vi "Launch NEW Window.vi"(5 "error in (no error)":errorcluster, 7 "Window Info":T1(array[cluster]), 8 "Window Type":T2, 9 "State Queue":string[](array[string])=["SC >>> Initialize"], 11 "wForms":waveform(dbl)[](array[waveform])) -> (19 "error OUT":errorcluster)   [LabVIEW 2020, in "SPWB.lvclass"]
uses:
  SPWB.lvclass
  Controls/Analysis Type.ctl
  API/GSwFormDSP_class/GSwFormDSP.lvclass
  <vilib>/addons/_AddQ/G#Object/G#Object.lvclass
panel:
  # "Please Wait ....\nOpening a NEW Window!"
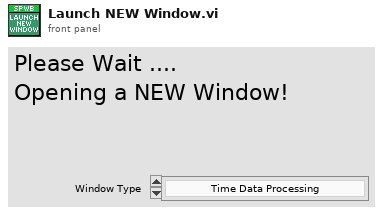
[diagram p1: front panel]
types:
  T1 = cluster{"Window Name Index":string, "wForm Ref":refnum<class "GSwFormDSP.lvclass">}[]
  T2 = typedef "SPWB.lvclass/Analysis Type.ctl" = enum16{"Time Data Processing", "FFT Analysis", "Time Frequency Analysis", "Transfer Functions"}
  T3 = cluster{"Window Name Index":string, "wForm Ref":refnum<class "GSwFormDSP.lvclass">}
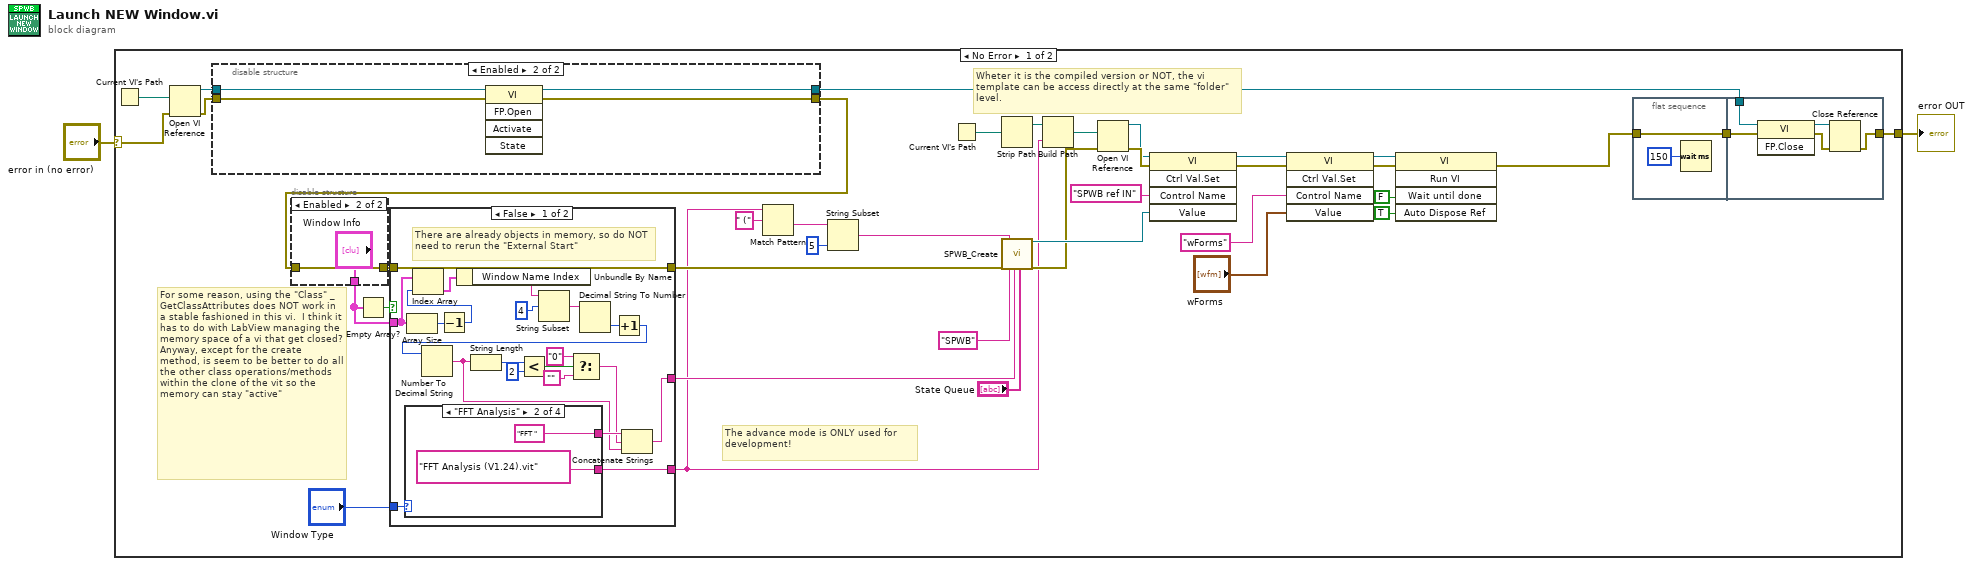
[diagram p0: block diagram]
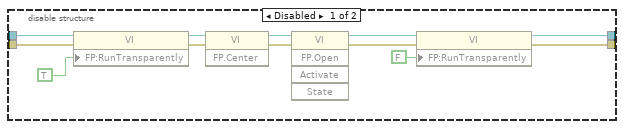
[diagram p2: hidden frame]
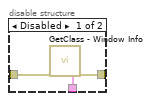
[diagram p3: hidden frame]
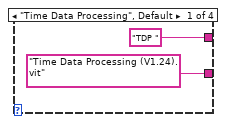
[diagram p4: hidden frame]
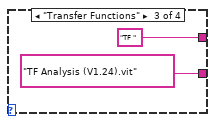
[diagram p5: hidden frame]
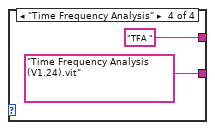
[diagram p6: hidden frame]
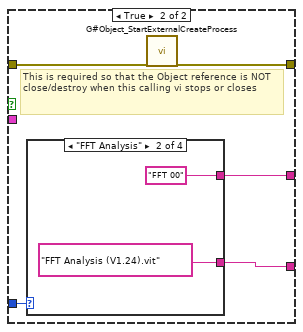
[diagram p7: hidden frame]
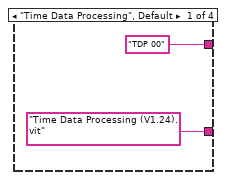
[diagram p8: hidden frame]
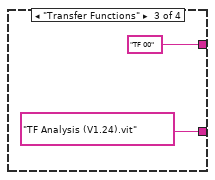
[diagram p9: hidden frame]
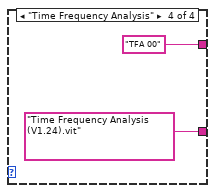
[diagram p10: hidden frame]
diagram:
  n1 = case shown="No Error" "error in (no error)" {
    selector: "error in (no error)" -> [w14 w111]
    tunnel: [w16 w111] -> w1
    frame No Error {
      # "The advance mode is ONLY used for development!"
      # "For some reason, using the \"Class\" _GetClassAttributes does NOT work in a stable fashioned in this vi.  I think it has to do with LabView managing the memory space of a vi that get closed?  Anyway, except for the create method, is seem to be better to do all the other class operations/methods within the clone of the vit so the memory can stay \"active\""
      # "Wheter it is the compiled version or NOT, the vi template can be access directly at the same \"folder\" level."
      n2 = Current VI's Path() -> (path=w15:path)
      n3 = Open VI Reference(vi path=w15, error in (no error)=w14) -> (vi reference=w7:refnum<vi>, error out=w6:errorcluster)  [unwired: 4 out]
      n4 = disable-structure shown="Enabled" {
        disable-tunnel: w7 -> [w49 w56]
        disable-tunnel: w6 -> [w47 w55]
        disable-tunnel: [w45 w54] -> w5
        disable-tunnel: [w42 w53] -> w4
        frame Disabled {
          n5 = property class="VI"(reference=w49, error in=w47, "FP:RunTransparently"=TRUE ("Front Panel Window:Run VI Transparently")) -> (reference out=w48:refnum<vi>, error out=w46:errorcluster)
          n6 = invoke class="VI" method="FP.Center"(reference=w48, error in=w46) -> (reference out=w52:refnum<vi>, error out=w51:errorcluster)  [unwired: 1 in, 1 out]
          n7 = invoke class="VI" method="FP.Open"(reference=w52, error in=w51) -> (reference out=w44:refnum<vi>, error out=w43:errorcluster)  [unwired: 3 in, 3 out]
          n8 = property class="VI"(reference=w44, error in=w43, "FP:RunTransparently"=FALSE ("Front Panel Window:Run VI Transparently")) -> (reference out=w45:refnum<vi>, error out=w42:errorcluster)
        }
        frame Enabled {
          n9 = invoke class="VI" method="FP.Open"(reference=w56, error in=w55) -> (reference out=w54:refnum<vi>, error out=w53:errorcluster)  [unwired: 3 in, 3 out]
        }
      }
      n10 = disable-structure shown="Enabled" {
        disable-tunnel: [w59 w61] -> w29
        disable-tunnel: [w58 "Window Info"] -> w26
        disable-tunnel: w4 -> [w57 w61]
        frame Disabled {
          n11 = call "GetClass - Window Info.vi"("error in (no error)"=w57) -> ("Window Info"=w58:T1, "error out"=w59:errorcluster)  [unwired: 17 in]
        }
        frame Enabled {
        }
      }
      n12 = Empty Array?(array=w26) -> (empty?=w30:bool)
      n13 = case shown="False" w30 {
        tunnel: [w89 w102] -> w25
        tunnel: w29 -> [w89 w101]
        tunnel: [w74 w100] -> w28
        tunnel: "Window Type" -> [w88 w99]
        tunnel: [w72 w98] -> w9
        tunnel: w26 -> [w73 _]
        frame False {
          # "There are already objects in memory, so do NOT need to rerun the \"External Start\""
          n14 = case shown="\"FFT Analysis\"" w88 {
            tunnel: ["Time Data Processing (V1.24).vit" ("name or relative path") "FFT Analysis (V1.24).vit" ("name or relative path") "TF Analysis (V1.24).vit" ("name or relative path") "Time Frequency Analysis (V1.24).vit" ("name or relative path")] -> w72
            tunnel: ["TDP " "FFT " "TF " "TFA "] -> w87
            frame "Time Data Processing", Default {
            }
            frame "FFT Analysis" {
            }
            frame "Transfer Functions" {
            }
            frame "Time Frequency Analysis" {
            }
          }
          n15 = Array Size(array=w73) -> (size(s)=w86:i32)
          n16 = Decrement(x=w86) -> (x-1=w71:i32)
          n17 = Index Array(array=w73, index=w71) -> (element=w70:T3)
          n18 = Unbundle By Name(w70) -> ("Window Name Index"=w69:string)
          n19 = String Subset(string=w69, offset (0)=4) -> (substring=w84:string)  [unwired: 1 in]
          n20 = Decimal String To Number(string=w84) -> (number=w83:i32)  [unwired: 2 in, 1 out]
          n21 = Increment(x=w83) -> (x+1=w77:i32)
          n22 = Number To Decimal String(number=w77) -> (decimal integer string=w76:string)  [unwired: 1 in]
          n23 = String Length(string=w76) -> (length=w78:i32)
          n24 = Less?(x=w78, y=2) -> (x < y?=w80:bool)
          n25 = Select(t="0", s=w80, f="") -> (s? t:f=w75:string)
          n26 = Concatenate Strings(w87, w75, w76) -> (w74:string)
        }
        frame True {
          # "This is required so that the Object reference is NOT close/destroy when this calling vi stops or closes"
          n27 = case shown="\"FFT Analysis\"" w99 {
            tunnel: ["Time Data Processing (V1.24).vit" ("name or relative path") "FFT Analysis (V1.24).vit" ("name or relative path") "TF Analysis (V1.24).vit" ("name or relative path") "Time Frequency Analysis (V1.24).vit" ("name or relative path")] -> w98
            tunnel: ["TDP 00" "FFT 00" "TF 00" "TFA 00"] -> w100
            frame "Time Data Processing", Default {
            }
            frame "FFT Analysis" {
            }
            frame "Transfer Functions" {
            }
            frame "Time Frequency Analysis" {
            }
          }
          n28 = call <vilib>:"G#Object_StartExternalCreateProcess.vi"("error in (no error)"=w101) -> ("error out"=w102:errorcluster)  [unwired: 18 in]
        }
      }
      n29 = Match Pattern(string=w9, regular expression=" (") -> (after substring=w11:string)  [unwired: 1 in, 3 out]
      n30 = String Subset(string=w11, length (rest)=5 ("length (rest)")) -> (substring=w8:string)  [unwired: 1 in]
      n31 = Current VI's Path() -> (path=w40:path)
      n32 = Strip Path(path=w40) -> (stripped path=w38:path)  [unwired: 1 out]
      n33 = call "SPWB_Create.vi"("error in (no error)"=w25, "Version #"=w8, "Application Name"="SPWB", "Window Name Index"=w28, "State Queue"="State Queue") -> ("reference out"=w31:refnum<class "SPWB.lvclass">, "error out"=w24:errorcluster)  [unwired: 13 in]
      n34 = Build Path(base path=w38, name or relative path=w9) -> (appended path=w39:path)
      n35 = Open VI Reference(vi path=w39, error in (no error)=w24) -> (vi reference=w35:refnum<vi>, error out=w36:errorcluster)  [unwired: 4 out]
      n36 = invoke class="VI" method="Ctrl Val.Set"(reference=w35, error in=w36, "Control Name"="SPWB ref IN", "Value"=w31) -> (reference out=w22:refnum<vi>, error out=w20:errorcluster)  [unwired: 1 in, 3 out]
      n37 = invoke class="VI" method="Ctrl Val.Set"(reference=w22, error in=w20, "Control Name"="wForms", "Value"="wForms") -> (reference out=w21:refnum<vi>, error out=w19:errorcluster)  [unwired: 1 in, 3 out]
      n38 = invoke class="VI" method="Run VI"(reference=w21, error in=w19, "Wait until done"=FALSE, "Auto Dispose Ref"=TRUE) -> (error out=w3:errorcluster)  [unwired: 1 in, 4 out]
      n39 = flat-sequence {
        tunnel: w3 -> [w63]
        tunnel: [w63] -> w13
        tunnel: [w65] -> w16
        tunnel: w5 -> [w68]
        tunnel: w13 -> [w64]
        frame #0 {
          n40 = Wait (ms)(milliseconds to wait=u32 150) -> ()  [unwired: 1 out]
        }
        frame #1 {
          n41 = invoke class="VI" method="FP.Close"(reference=w68, error in=w64) -> (reference out=w66:refnum<vi>, error out=w67:errorcluster)  [unwired: 1 in, 1 out]
          n42 = Close Reference(reference=w66, error in (no error)=w67) -> (error out=w65:errorcluster)
        }
      }
    }
    frame Error {
    }
  }
  "error OUT" <- w1
